vi "Locate edges.vi"(6 "Seen last value":bool, 9 "Last value":i32, 10 "First value":i32, 11 "Values":i32[](array[numeric])) -> (3 "Edge indexies":i32[](array[numeric]), 4 "Seen last value out":bool)   [LabVIEW 2016]
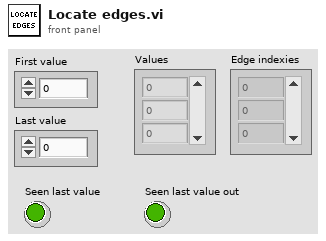
[diagram p1: front panel]
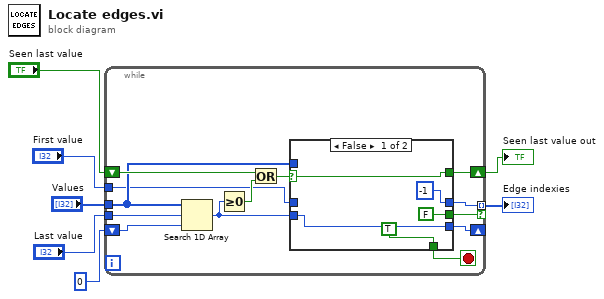
[diagram p0: block diagram]
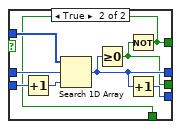
[diagram p2: hidden frame]
diagram:
  n1 = while {
    tunnel: "Last value" -> [w20]
    tunnel: "Values" -> [w16]
    tunnel: "First value" -> [w14]
    shift-right: [w9] -> w1
    shift-left: "Seen last value" -> [w18]
    tunnel: [w13] -> w2 mode=indexing if=w12
    shift-right: [w10] -> _
    shift-left: 0 -> [w11]
    stop <- w8 stop-if-true
    n2 = Search 1D Array(1D array=w16, element=w20, start index (0)=w11) -> (index of element=w15:i32)
    n3 = Greater Or Equal To 0?(x=w15) -> (x >= 0?=w19:bool)
    n4 = Or(x=w18, y=w19) -> (x .or. y?=w17:bool)
    n5 = case shown="False" w17 {
      selector: w17 -> [w22 _]
      tunnel: w16 -> [_ w33]
      tunnel: w15 -> [w23 w31]
      tunnel: w14 -> [_ w30]
      tunnel: [-1 ("index of element") w28] -> w13
      tunnel: [FALSE w27] -> w12
      tunnel: [w23 w29] -> w10
      tunnel: [w22 w26] -> w9
      tunnel: [TRUE w26] -> w8
      frame False {
      }
      frame True {
        n6 = Increment(x=w31) -> (x+1=w32:i32)
        n7 = Search 1D Array(1D array=w33, element=w30, start index (0)=w32) -> (index of element=w28:i32)
        n8 = Greater Or Equal To 0?(x=w28) -> (x >= 0?=w27:bool)
        n9 = Not(x=w27) -> (.not. x?=w26:bool)
        n10 = Increment(x=w28) -> (x+1=w29:i32)
      }
    }
  }
  "Seen last value out" <- w1
  "Edge indexies" <- w2
